vi "modbus slave new.vi"() -> ()   [LabVIEW 2016]
uses:
  <vilib>/NI/Modbus Library/API/Wrapper/Create TCP Slave.vi
  <vilib>/NI/Modbus Library/API/slave/Modbus Slave.lvclass
  <vilib>/NI/Modbus Library/API/Wrapper/API Main.lvlib
  <vilib>/ptbypt/NI_PtbyPt.lvlib
panel:
  out "读取register values 2":u16[](array[numeric])
  out "status":bool
  in  "写入registers to write":u16[](array[numeric])
  out "读取register values":u16[](array[numeric])
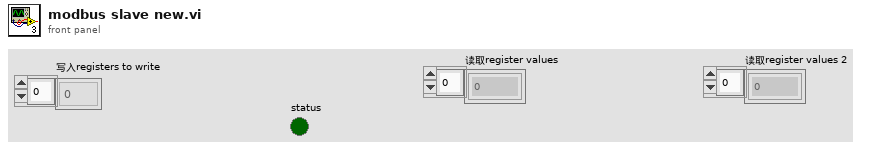
[diagram p1: front panel]
types:
  T1 = enum16{"", "CODMn", "PH", "氨氮", "总氮", "总磷", "CODCr", "电导率", "水温", "溶解氧", "浊度", "叶绿素", "藻密度", "ORP"}
  T2 = enum16{"i13001", "i13002", "i13003", "i13004", "i13005", "i13006", "i13007", "i13008", "i13009", "i13010", "i13011", "i13012", "i13013", "i13014", "i13015", "i13016", "i13017", "i13101", "i13102", "i13103", "i13104", "i13105", "i13106", "i13107", "i13108", "i13109", "i13110"}
  T3 = enum16{"启动整机", "停止整机", "标样核查", "加标回收", "平行样测试", "零点核查", "跨度核查", "校零", "校标"}
  T4 = cluster{"status":bool, "代码":u16, "source":string}
  T5 = cluster{"系统时间":timestamp, "工作状态":u16, "测量模式":enum16{"待机", "连续模式", "周期模式", "定点模式", "受控模式", "手动模式"}, "告警代码":u16, "故障代码":u16, "日志代码":u16, "软件版本":u16, "F0":sgl, "F1":sgl, "F2":sgl, "F3":sgl, "T":sgl, "H":sgl, "id":u16, "flowid":u16, "量程":u16, "总磷控温温度1":sgl, "营养盐控温温度2":sgl, "ADC":sgl}
  T6 = cluster{"系统时间":timestamp, "工作状态":u16, "测量模式":enum16{"待机", "连续模式", "周期模式", "定点模式", "受控模式", "手动模式"}, "告警代码":u16, "故障代码":u16, "日志代码":u16, "软件版本":u16, "A":sgl, "B":sgl, "K":sgl, "当前滴定数":sgl, "T":sgl, "H":sgl, "id":u16, "flowid":u16, "量程":u16, "加热实时温度":sgl, "当前ORP值":sgl, "运行时间":sgl, "当前步骤剩余时间":sgl, "结束滴定数":sgl, "注射泵保温温度":sgl, "匹配滴定数X0":u16, "X^2":sgl, "X":sgl, "B 2":sgl}
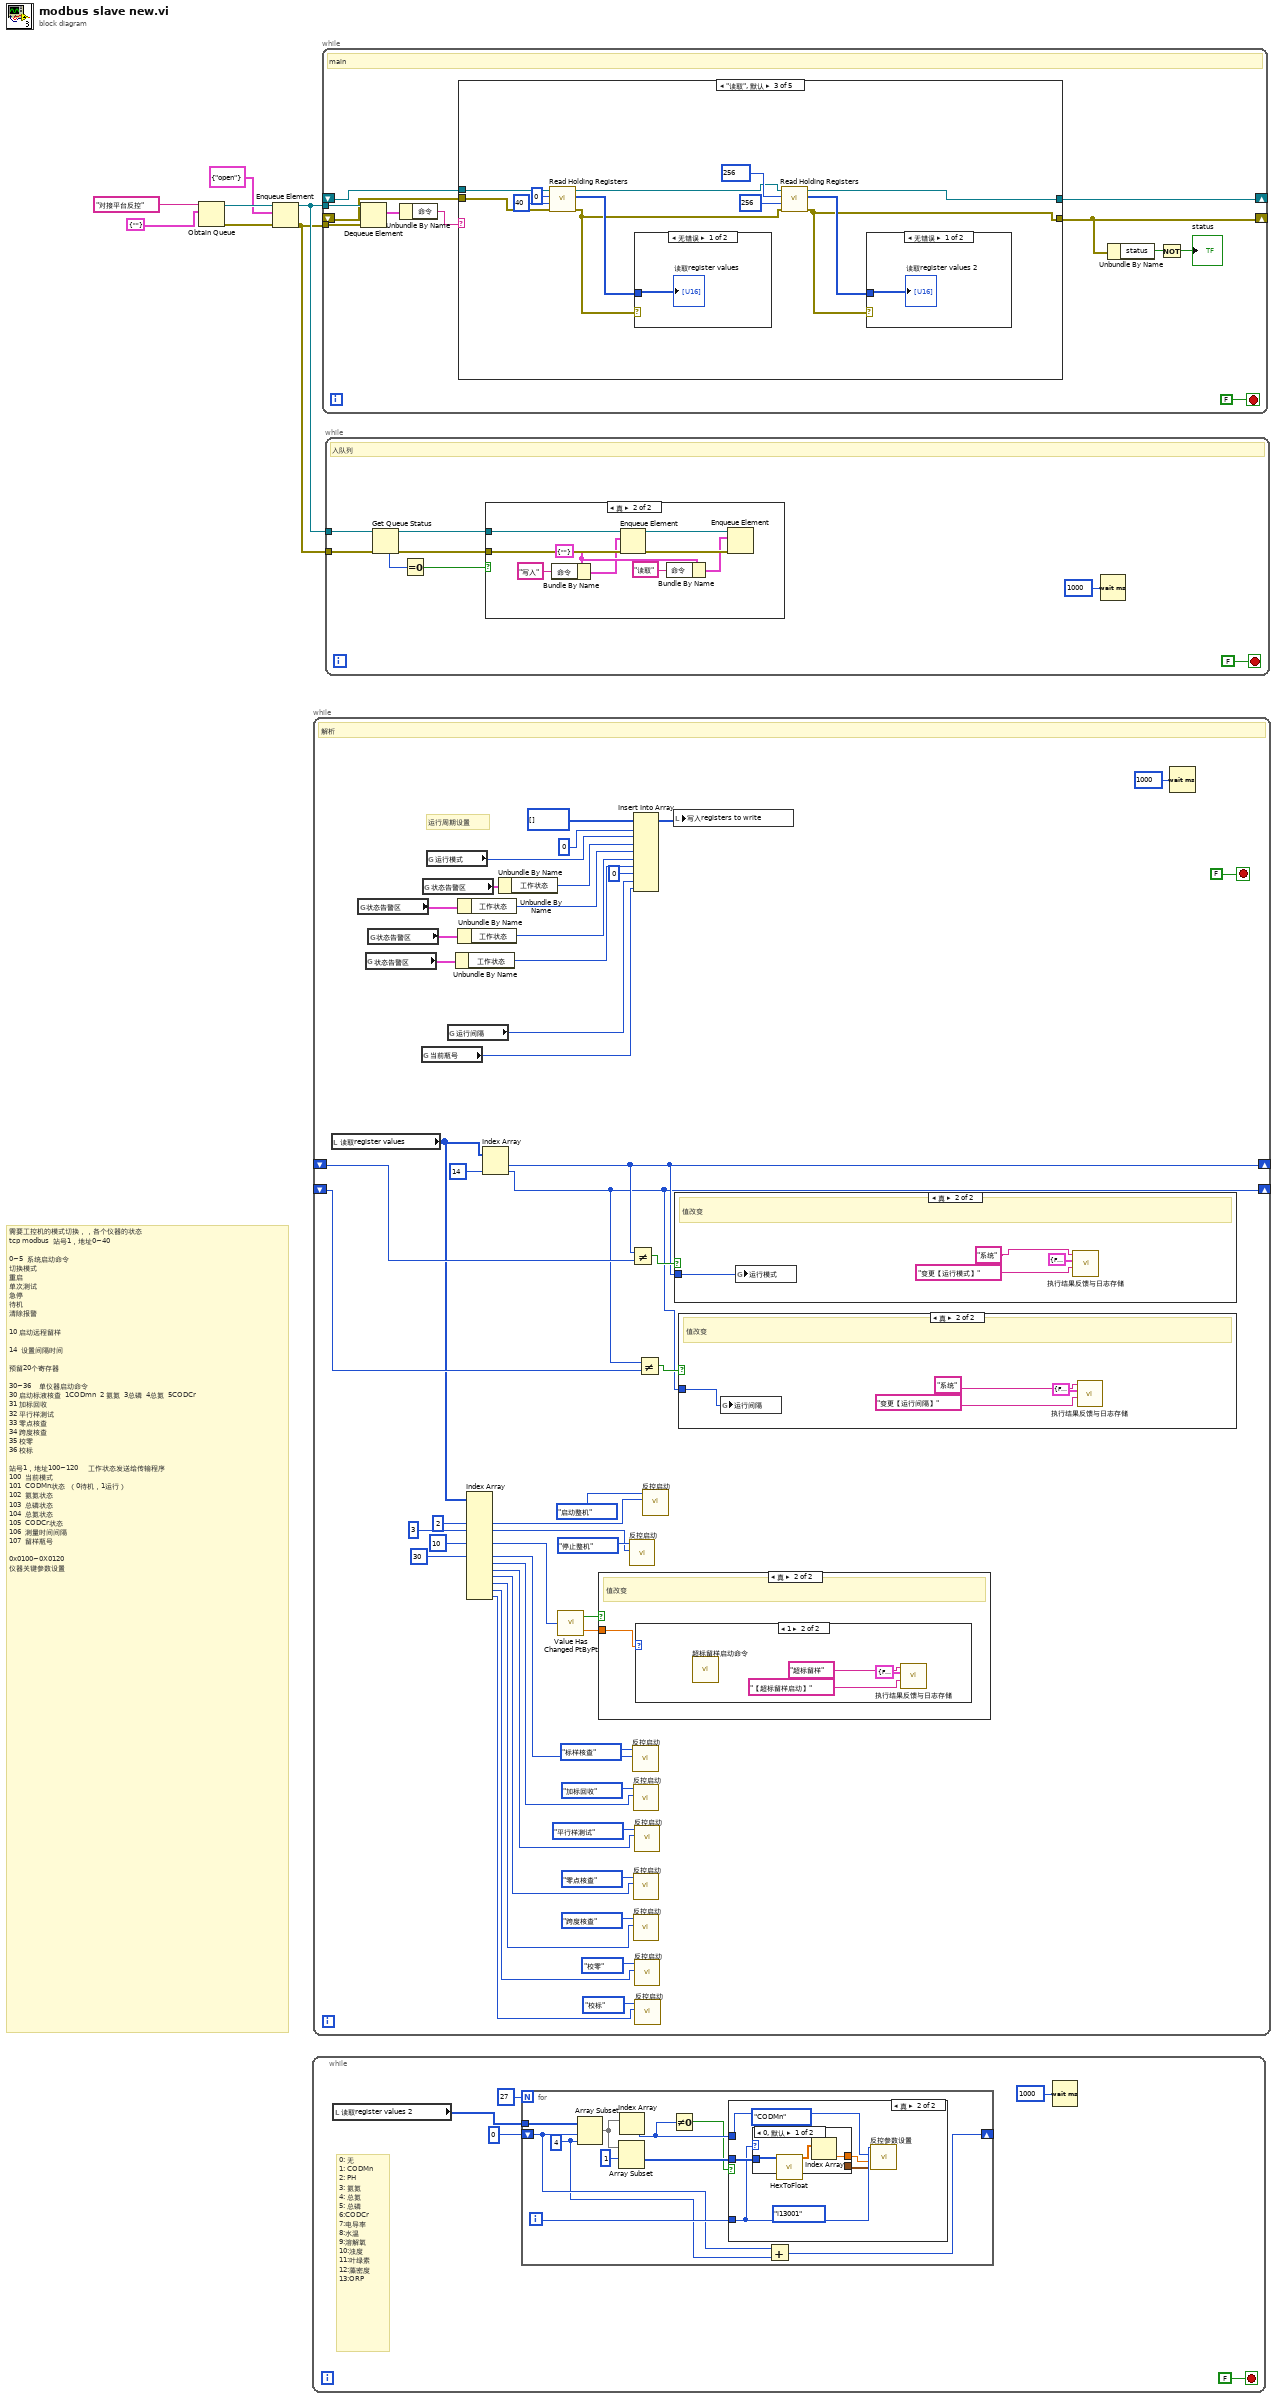
[diagram p0: block diagram]
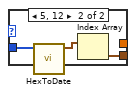
[diagram p3: hidden frame]
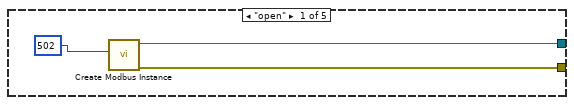
[diagram p9: hidden frame]
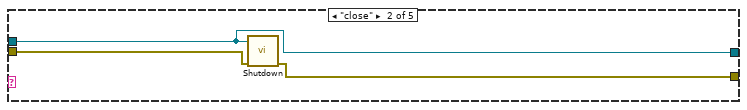
[diagram p10: hidden frame]
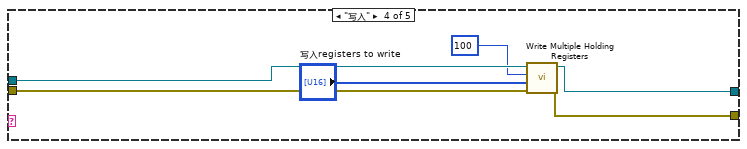
[diagram p13: hidden frame]
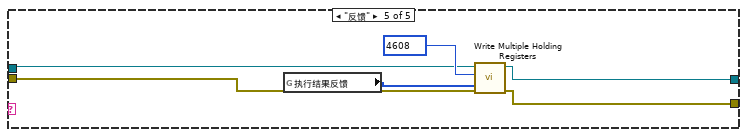
[diagram p14: hidden frame]
diagram:
  # "需要工控机的模式切换，，各个仪器的状态\ntcp modbus  站号1，地址0~40\n\n0~5  系统启动命令\n切换模式\n重启\n单次测试\n急停\n待机\n清除报警\n\n10 启动远程留样\n\n14  设置间隔时间\n\n预留20个寄存器\n\n30~36    单仪器启动命令\n30 启动标液核查  1CODmn  2 氨氮  3总磷  4总氮  5CODCr\n31 加标回收\n32 平行样测试\n33 零点核查\n34 跨度核查\n35 校零\n36 校标\n\n站号1，地址100~120     工作状态发送给传输程序\n100  当前模式\n101  CODMn状态  （0待机，1运行）\n102  氨氮状态\n103  总磷状态\n104  总氮状态\n105  CODCr状态\n106  测量时间间隔\n107  留样瓶号\n\n0x0100~0X0120\n仪器关键参数设置"
  n1 = Obtain Queue(name (unnamed)="对接平台反控" ("名称（未命名）"), element data type=cluster{"命令":string} {"命令"=""}) -> (queue out=w5:refnum<queue>, error out=w4:errorcluster)  [unwired: 3 in, 1 out]
  n2 = Enqueue Element(queue=w5, element=cluster{"命令":string} {"命令"="open"} ("元素"), error in (no error)=w4) -> (queue out=w2:refnum<queue>, error out=w1:errorcluster)  [unwired: 1 in, 1 out]
  n3 = while {
    stop <- FALSE stop-if-true
    # "0: 无\n1: CODMn\n2: PH\n3: 氨氮\n4: 总氮\n5: 总磷\n6:CODCr\n7:电导率\n8:水温\n9:溶解氧\n10:浊度\n11:叶绿素\n12:藻密度\n13:ORP"
    n4 = local read "读取register values 2"() -> (w10:u16[])
    n5 = for {
      N: 27 -> [_]
      tunnel: w10 -> [w22]
      shift-right: [w13] -> _
      shift-left: 0 ("索引") -> [w15]
      i -> [w18]
      w14 = 4 ("长度")
      n6 = Array Subset(array=w22, index=w15, length=w14) -> (w21:u16[])
      n7 = Array Subset(array=w21, index=1 ("索引")) -> (w19:u16[])  [unwired: 1 in]
      n8 = Index Array(array=w21) -> (element=w17:u16)  [unwired: 1 in]
      n9 = Not Equal To 0?(x=w17) -> (x != 0?=w16:bool)
      n10 = case shown="真" w16 {
        tunnel: w19 -> [_ w27]
        tunnel: w18 -> [_ w26]
        tunnel: w17 -> [_ w25]
        frame False {
        }
        frame True {
          (unwired) T1."CODMn"
          (unwired) T2."i13001" ("设置类型")
          n11 = case shown="0, 默认" w26 {
            tunnel: w27 -> [w30 w33]
            tunnel: [_ w31] -> w23
            tunnel: [w28 _] -> w24
            frame 0, Default {
              n12 = call "HexToFloat.vi"("数组"=w30) -> ("FLOAT"=w29:sgl[])  [unwired: 10 in]
              n13 = Index Array(array=w29) -> (element=w28:sgl)  [unwired: 1 in]
            }
            frame 5, 12 {
              n14 = call "HexToDate.vi"("数组"=w33) -> ("DATE"=w32:timestamp[])  [unwired: 10 in]
              n15 = Index Array(array=w32) -> (element=w31:timestamp)  [unwired: 1 in]
            }
          }
          n16 = call "反控参数设置.vi"("value time"=w23, "value float"=w24, "设置参数"=w25, "设置类型"=w26) -> ()  [unwired: 8 in]
        }
      }
      n17 = Add(x=w15, y=w14) -> (x+y=w13:i32)
    }
    n18 = Wait (ms)(milliseconds to wait=u32 1000 ("等待时间（毫秒）")) -> ()  [unwired: 1 out]
  }
  n19 = while {
    shift-right: [w67] -> _
    shift-left: _ -> [w69]
    shift-right: [w64] -> _
    shift-left: _ -> [w66]
    stop <- FALSE stop-if-true
    # "运行周期设置"
    # "解析"
    n20 = local read "读取register values"() -> (w59:u16[])
    n21 = global read "VAR总磷总氮全局变量.vi" "状态告警区"() -> (w78:T5)
    n22 = global read "VAR总磷总氮全局变量.vi" "状态告警区"() -> (w74:T5)
    n23 = global read "VAR总磷总氮全局变量.vi" "状态告警区"() -> (w76:T5)
    n24 = global read "外部交互全局.vi" "当前瓶号"() -> (w37:u16)
    n25 = global read "VARCODMn全局变量.vi" "状态告警区"() -> (w36:T6)
    n26 = global read "系统设置全局变量.vi" "运行模式"() -> (w80:enum16{"维护模式", "常规模式", "应急模式", "质控模式"})
    n27 = global read "系统设置全局变量.vi" "运行间隔"() -> (w72:i16)
    n28 = Unbundle By Name(w74) -> ("工作状态"=w73:u16)
    n29 = Unbundle By Name(w78) -> ("工作状态"=w77:u16)
    n30 = Unbundle By Name(w76) -> ("工作状态"=w75:u16)
    n31 = Index Array(array=w59, index #3=2 ("索引"), index #4=3 ("索引"), index #6=10 ("索引"), index #8=30 ("索引")) -> (element #3=w58:u16, element #4=w55:u16, element #6=w52:u16, element #8=w50:u16, element #9=w44:u16, element #10=w43:u16, element #11=w42:u16, element #12=w40:u16, element #13=w39:u16, element #14=w38:u16)  [unwired: 10 in, 4 out]
    n32 = Index Array(array=w59, index #2=14 ("索引")) -> (element #1=w67:u16, element #2=w64:u16)  [unwired: 1 in]
    n33 = Unbundle By Name(w36) -> ("工作状态"=w35:u16)
    n34 = call <vilib>:"Value Has Changed PtByPt.vi"("input data point"=w52) -> ("has changed"=w54:bool, "output data point"=w53:dbl)  [unwired: 1 in]
    n35 = case shown="真" w54 {
      tunnel: w53 -> [_ w84]
      frame False {
      }
      frame True {
        # "值改变"
        n36 = case shown="1" w84 {
          frame 0, Default {
          }
          frame 1 {
            n37 = call "超标留样启动命令.vi"() -> ()  [unwired: 12 in]
            n38 = call "执行结果反馈与日志存储.vi"("日志信息"="【超标留样启动】", "error out"=T4 {"status"=FALSE, "代码"=1, "source"=""}, "设备"="超标留样") -> ()  [unwired: 9 in]
          }
        }
      }
    }
    n39 = call "反控启动.vi"("启动参数"=w55, "启动类型"=T3."停止整机") -> ()  [unwired: 10 in]
    n40 = Not Equal?(x=w67, y=w69) -> (x != y?=w68:bool)
    n41 = call "反控启动.vi"("启动参数"=w50, "启动类型"=T3."标样核查") -> ()  [unwired: 10 in]
    n42 = Insert Into Array(array=u16[] [] ("values to write"), index=0 ("索引"), new element #1=w80, new element #2=w35, new element #3=w77, new element #4=w75, new element #5=w73, new element #6=u16 0 ("新元素/子数组"), new element #7=w72, new element #8=w37) -> (w71:u16[])
    n43 = call "反控启动.vi"("启动参数"=w44, "启动类型"=T3."加标回收") -> ()  [unwired: 10 in]
    n44 = call "反控启动.vi"("启动参数"=w42, "启动类型"=T3."零点核查") -> ()  [unwired: 10 in]
    n45 = call "反控启动.vi"("启动参数"=w40, "启动类型"=T3."跨度核查") -> ()  [unwired: 10 in]
    n46 = call "反控启动.vi"("启动参数"=w43, "启动类型"=T3."平行样测试") -> ()  [unwired: 10 in]
    n47 = call "反控启动.vi"("启动参数"=w39, "启动类型"=T3."校零") -> ()  [unwired: 10 in]
    n48 = call "反控启动.vi"("启动参数"=w38, "启动类型"=T3."校标") -> ()  [unwired: 10 in]
    n49 = Not Equal?(x=w64, y=w66) -> (x != y?=w65:bool)
    n50 = call "反控启动.vi"("启动参数"=w58, "启动类型"=T3."启动整机") -> ()  [unwired: 10 in]
    n51 = local write "写入registers to write"(w71) -> ()
    n52 = case shown="真" w68 {
      tunnel: w67 -> [_ w95]
      frame False {
      }
      frame True {
        # "值改变"
        n53 = global write "系统设置全局变量.vi" "运行模式"(w95) -> ()
        n54 = call "执行结果反馈与日志存储.vi"("日志信息"="变更【运行模式】", "error out"=T4 {"status"=FALSE, "代码"=1, "source"=""}, "设备"="系统") -> ()  [unwired: 9 in]
      }
    }
    n55 = case shown="真" w65 {
      tunnel: w64 -> [_ w91]
      frame False {
      }
      frame True {
        # "值改变"
        n56 = global write "系统设置全局变量.vi" "运行间隔"(w91) -> ()
        n57 = call "执行结果反馈与日志存储.vi"("日志信息"="变更【运行间隔】", "error out"=T4 {"status"=FALSE, "代码"=1, "source"=""}, "设备"="系统") -> ()  [unwired: 9 in]
      }
    }
    n58 = Wait (ms)(milliseconds to wait=u32 1000 ("等待时间（毫秒）")) -> ()  [unwired: 1 out]
  }
  n59 = while {
    tunnel: w2 -> [w106]
    tunnel: w1 -> [w105]
    shift-right: [w102] -> _
    shift-left: _ -> [w101]
    shift-right: [w96] -> _
    shift-left: _ -> [w100]
    stop <- FALSE stop-if-true
    # "main"
    n60 = Dequeue Element(queue=w106, error in (no error)=w105) -> (element=w104:cluster{"命令":string})  [unwired: 1 in, 3 out]
    n61 = Unbundle By Name(w104) -> ("命令"=w103:string)
    n62 = case shown="\"读取\", 默认" w103 {
      tunnel: [w107 w110 w114 w128 w135] -> w102
      tunnel: [w108 w111 w113 w127 w134] -> w96
      tunnel: w101 -> [_ w110 w124 w132 w137]
      tunnel: w100 -> [_ w112 w123 w131 w136]
      frame "open" {
        n63 = call-poly <vilib>:"Create Modbus Instance.vi"("port (502)"=u16 502) -> ("error out"=w108:errorcluster, "TCP slave instance"=w107:refnum<class "Modbus Slave.lvclass">)  [unwired: 9 in]
      }
      frame "close" {
        n64 = call-dynamic "Shutdown.vi"("error in"=w112, "Modbus slave in"=w110) -> ("error out"=w111:errorcluster)  [unwired: 9 in]
      }
      frame "读取", Default {
        n65 = call-dynamic "Read Holding Registers.vi"("error in"=w123, "number of inputs"=u16 40, "starting address"=u16 0, "Modbus slave in"=w124) -> ("error out"=w115:errorcluster, "register values"=w120:u16[], "Modbus slave out"=w116:refnum<class "Modbus Slave.lvclass">)  [unwired: 5 in]
        n66 = case shown="无错误" w115 {
          tunnel: w120 -> [w126 _]
          frame No Error {
            "读取register values" <- w126
          }
          frame Error {
          }
        }
        n67 = call-dynamic "Read Holding Registers.vi"("error in"=w115, "number of inputs"=u16 256, "starting address"=u16 256, "Modbus slave in"=w116) -> ("error out"=w113:errorcluster, "register values"=w119:u16[], "Modbus slave out"=w114:refnum<class "Modbus Slave.lvclass">)  [unwired: 5 in]
        n68 = case shown="无错误" w113 {
          tunnel: w119 -> [w125 _]
          frame No Error {
            "读取register values 2" <- w125
          }
          frame Error {
          }
        }
      }
      frame "写入" {
        n69 = call-dynamic "Write Multiple Holding Registers.vi"("error in"=w131, "registers to write"="写入registers to write", "starting address"=u16 100, "Modbus slave in"=w132) -> ("error out"=w127:errorcluster, "Modbus slave out"=w128:refnum<class "Modbus Slave.lvclass">)  [unwired: 6 in]
      }
      frame "反馈" {
        n70 = global read "modbus slave全局.vi" "执行结果反馈"() -> (w133:u16[])
        n71 = call-dynamic "Write Multiple Holding Registers.vi"("error in"=w136, "registers to write"=w133, "starting address"=u16 4608, "Modbus slave in"=w137) -> ("error out"=w134:errorcluster, "Modbus slave out"=w135:refnum<class "Modbus Slave.lvclass">)  [unwired: 6 in]
      }
    }
    n72 = Unbundle By Name(w96) -> ("status"=w98:bool)
    n73 = Not(x=w98) -> (.not. x?=→"status":bool)
  }
  n74 = while {
    tunnel: w2 -> [w146]
    tunnel: w1 -> [w144]
    stop <- FALSE stop-if-true
    # "入队列"
    n75 = Get Queue Status(queue=w146, error in (no error)=w144) -> (queue out=w145:refnum<queue>, error out=w143:errorcluster, # elements in queue=w142:i32)  [unwired: 1 in, 5 out]
    n76 = Equal To 0?(x=w142) -> (x = 0?=w141:bool)
    n77 = case shown="真" w141 {
      tunnel: w145 -> [_ w155]
      tunnel: w143 -> [_ w154]
      frame False {
      }
      frame True {
        w150 = cluster{"命令":string} {"命令"=""} ("元素")
        n78 = Bundle By Name(cluster=w150, "命令"="写入") -> (w149:cluster{"命令":string})
        n79 = Enqueue Element(queue=w155, element=w149, error in (no error)=w154) -> (queue out=w153:refnum<queue>, error out=w152:errorcluster)  [unwired: 1 in, 1 out]
        n80 = Bundle By Name(cluster=w150, "命令"="读取") -> (w147:cluster{"命令":string})
        n81 = Enqueue Element(queue=w153, element=w147, error in (no error)=w152) -> ()  [unwired: 1 in, 3 out]
      }
    }
    n82 = Wait (ms)(milliseconds to wait=u32 1000 ("等待时间（毫秒）")) -> ()  [unwired: 1 out]
  }
